vi "简易温度转换器（利用单位）.vi"() -> ()   [LabVIEW 2012]
panel:
  in  "停止":bool
  in  "转换模式":T1(ring)
  in  "输入温度":dbl(slide) scale=-300.0..300.0
  out "转换温度":dbl(slide) scale=-300.0..300.0
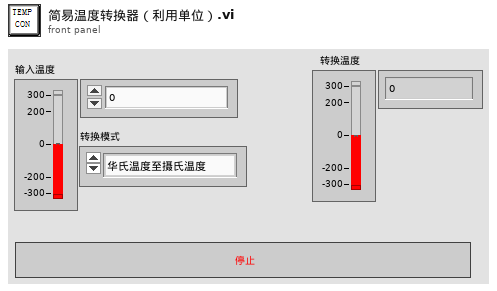
[diagram p1: front panel]
types:
  T1 = enum16{"华氏温度至摄氏温度", "摄氏温度至华氏温度", "开氏温度至摄氏温度", "摄氏温度至开氏温度", "开氏温度至华氏温度", "华氏温度至开氏温度"}
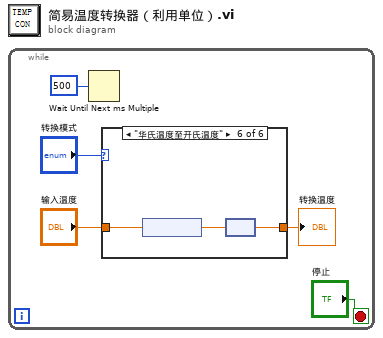
[diagram p0: block diagram]
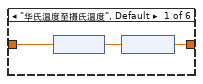
[diagram p2: hidden frame]
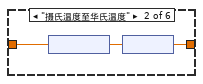
[diagram p3: hidden frame]
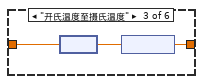
[diagram p4: hidden frame]
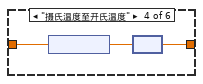
[diagram p5: hidden frame]
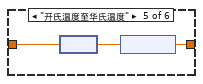
[diagram p6: hidden frame]
diagram:
  n1 = while {
    stop <- "停止" stop-if-true
    n2 = Wait Until Next ms Multiple(millisecond multiple=u32 500 ("毫秒倍数")) -> ()  [unwired: 1 out]
    n3 = case shown="\"华氏温度至开氏温度\"" "转换模式" {
      tunnel: "输入温度" -> [w8 w11 w14 w17 w20 w23]
      tunnel: [w6 w9 w12 w15 w18 w21] -> w1
      frame "华氏温度至摄氏温度", Default {
        n4 = node(w8) -> (w7:dbl[unit])
        n5 = node(w7) -> (w6:dbl)
      }
      frame "摄氏温度至华氏温度" {
        n6 = node(w11) -> (w10:dbl[unit])
        n7 = node(w10) -> (w9:dbl)
      }
      frame "开氏温度至摄氏温度" {
        n8 = node(w14) -> (w13:dbl[unit])
        n9 = node(w13) -> (w12:dbl)
      }
      frame "摄氏温度至开氏温度" {
        n10 = node(w17) -> (w16:dbl[unit])
        n11 = node(w16) -> (w15:dbl)
      }
      frame "开氏温度至华氏温度" {
        n12 = node(w20) -> (w19:dbl[unit])
        n13 = node(w19) -> (w18:dbl)
      }
      frame "华氏温度至开氏温度" {
        n14 = node(w23) -> (w22:dbl[unit])
        n15 = node(w22) -> (w21:dbl)
      }
    }
    "转换温度" <- w1
  }
